vi "dfd_X Equal Y (Array).vi"(0 "x":dbl[](array[numeric]), 3 "y":dbl[](array[numeric]), 4 "esp":dbl=1e-12) -> (6 "x = y?":bool)   [LabVIEW 2017, in "NI_DigFilterLicensed.lvlib"]
uses:
  <vilib>/addons/Digital Filter Design/NI_DigFilterLicensed.lvlib
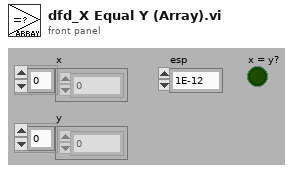
[diagram p1: front panel]
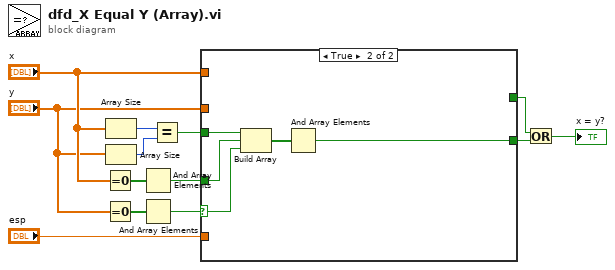
[diagram p0: block diagram]
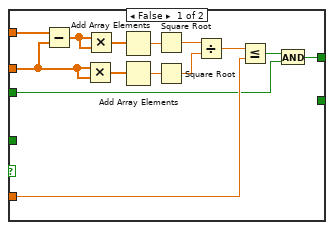
[diagram p2: hidden frame]
diagram:
  n1 = Equal To 0?(x="x") -> (x = 0?=w11:bool[])
  n2 = Equal To 0?(x="y") -> (x = 0?=w10:bool[])
  n3 = Array Size(array="x") -> (size(s)=w13:i32)
  n4 = Array Size(array="y") -> (size(s)=w12:i32)
  n5 = And Array Elements(Boolean array=w11) -> (logical AND=w7:bool)
  n6 = And Array Elements(Boolean array=w10) -> (logical AND=w8:bool)
  n7 = Equal?(x=w13, y=w12) -> (x = y?=w6:bool)
  n8 = case shown="True" w8 {
    selector: w8 -> [_ w29]
    tunnel: w7 -> [_ w30]
    tunnel: w6 -> [w15 w31]
    tunnel: "x" -> [w19 _]
    tunnel: "y" -> [w18 _]
    tunnel: "esp" -> [w17 _]
    tunnel: [_ w28] -> w2
    tunnel: [w14 _] -> w1
    frame False {
      n9 = Subtract(x=w19, y=w18) -> (x-y=w20:dbl[])
      n10 = Multiply(x=w18, y=w18) -> (x*y=w24:dbl[])
      n11 = Multiply(x=w20, y=w20) -> (x*y=w21:dbl[])
      n12 = Add Array Elements(numeric array=w21) -> (sum=w22:dbl)
      n13 = Add Array Elements(numeric array=w24) -> (sum=w25:dbl)
      n14 = Square Root(x=w22) -> (sqrt(x)=w23:dbl)
      n15 = Square Root(x=w25) -> (sqrt(x)=w26:dbl)
      n16 = Divide(x=w23, y=w26) -> (x/y=w27:dbl)
      n17 = Less Or Equal?(x=w27, y=w17) -> (x <= y?=w16:bool)
      n18 = And(x=w16, y=w15) -> (x .and. y?=w14:bool)
    }
    frame True {
      n19 = Build Array(w31, w30, w29) -> (w32:bool[])
      n20 = And Array Elements(Boolean array=w32) -> (logical AND=w28:bool)
    }
  }
  n21 = Or(x=w1, y=w2) -> (x .or. y?=→"x = y?":bool)
